vi "mqttWillWrite.vi"(8 "error in (no error)":errorcluster, 10 "Will Info":T1={"Will message"="Last Will", "Will Topic"="Will Topic"}, 11 "mqtt in":refnum<class "mqtt.lvclass">) -> (0 "error out":errorcluster, 3 "mqtt out":refnum<class "mqtt.lvclass">)   [LabVIEW 2015, in "mqtt.lvclass"]
uses:
  mqtt.lvclass
  mqttTypedef/mqttUserInformation.ctl
  mqtt.lvclass/mqtt.ctl
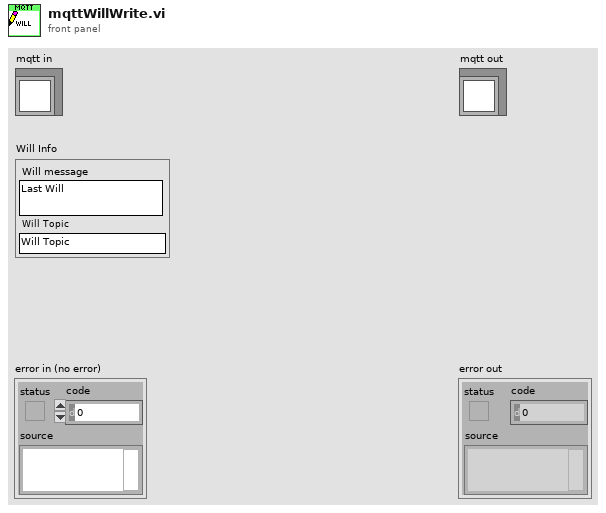
[diagram p1: front panel]
types:
  T1 = typedef "mqttUserInformation.ctl" = cluster{"Will message":string, "Will Topic":string}
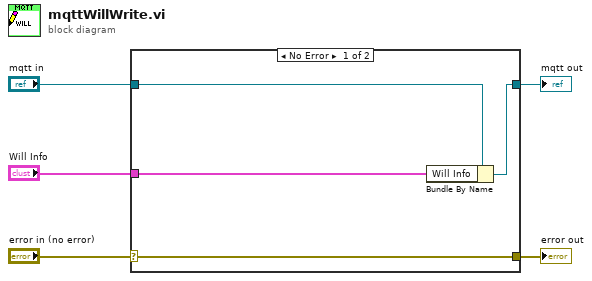
[diagram p0: block diagram]
diagram:
  n1 = case shown="No Error" "error in (no error)" {
    selector: "error in (no error)" -> [w9 w10]
    tunnel: [w9 w10] -> w4
    tunnel: [w7 w11] -> w2
    tunnel: "mqtt in" -> [w8 w11]
    tunnel: "Will Info" -> [w6 _]
    frame No Error {
      n2 = Bundle By Name(cluster=w8, "Will Info"=w6) -> (w7:refnum<class "mqtt.lvclass">)
    }
    frame Error {
    }
  }
  "error out" <- w4
  "mqtt out" <- w2
